vi "turn_back2.vi"(6 "Parâmetros Ini 2":T2={"Gyro Port"=0, "Sensor - Left"=3, "Sensor - Right"=2, "     Color \nSensor Port"=1, "Kp Front"=0.5, "Motor speed"=-15, "Distance to street"=0.0, "Motor speed turns"=16, "Kp Curvas"=0.0} {"Kp Front" format="%.3f"; "Color \nSensor Port" items=["Port 1", "Port 2", "Port 3", "Port 4"]; "Sensor - Right" items=["Port 1", "Port 2", "Port 3", "Port 4"]; "Sensor - Left" items=["Port 1", "Port 2", "Port 3", "Port 4"]; "Gyro Port" items=["Port 1", "Port 2", "Port 3", "Port 4"]}, 8 "NXT/EV3":T1) -> (1 "NXT/EV3 2":T1)   [LabVIEW 2016]
uses:
  <vilib>/NXT/Subs/LVHSConnector.ctl
  <vilib>/NXT/LegoClasses/BrickReference/BrickReference.lvclass
  parametros.ctl
  <vilib>/NXT/Block Support/NXT_InputPort.ctl
  <vilib>/NXT/Block Support/NXT_OutputPort.ctl
  <vilib>/NXT/Dual Mode Library/Sensors/EV3_Gyro_Angle.vi
  <vilib>/NXT/NXTIO Xnodes/NXTIONodeSubVIs/NXTMoveMotors.vi
  <vilib>/NXT/NXTIO Xnodes/NXTIONodeSubVIs/NXTStopMotors.vi
  <vilib>/NXT/NXTIO Xnodes/AddressXNode/NXTIOAddress.xnode
  <vilib>/NXT/NXTIO Xnodes/NXTIOXNode/NXTIO.xnode
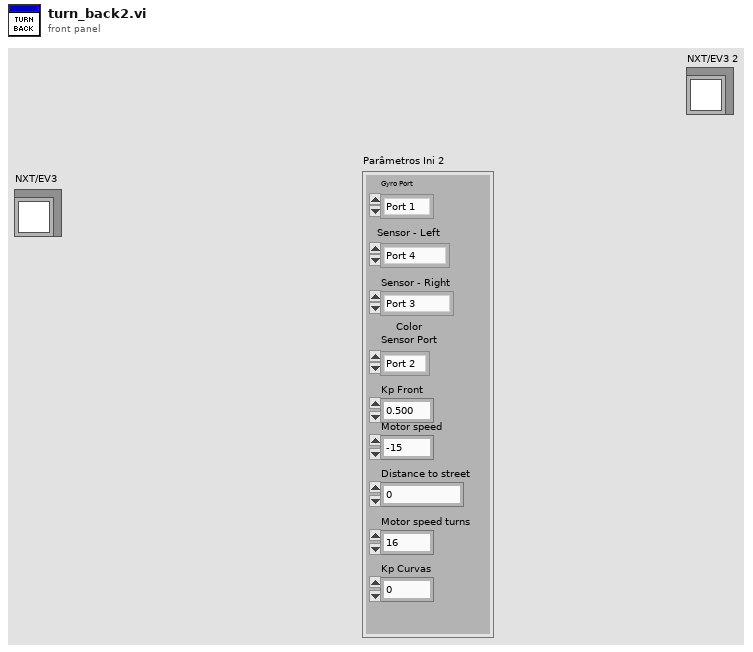
[diagram p1: front panel]
types:
  T1 = typedef "LVHSConnector.ctl" = refnum<class "BrickReference.lvclass">
  T2 = typedef "parametros.ctl" = cluster{"Gyro Port":T3, "Sensor - Left":T3, "Sensor - Right":T3, "     Color \nSensor Port":T3, "Kp Front":dbl, "Motor speed":i32, "Distance to street":dbl, "Motor speed turns":i32, "Kp Curvas":dbl}
  T3 = typedef "NXT_InputPort.ctl" = u32
  T4 = typedef "NXT_OutputPort.ctl" = u8
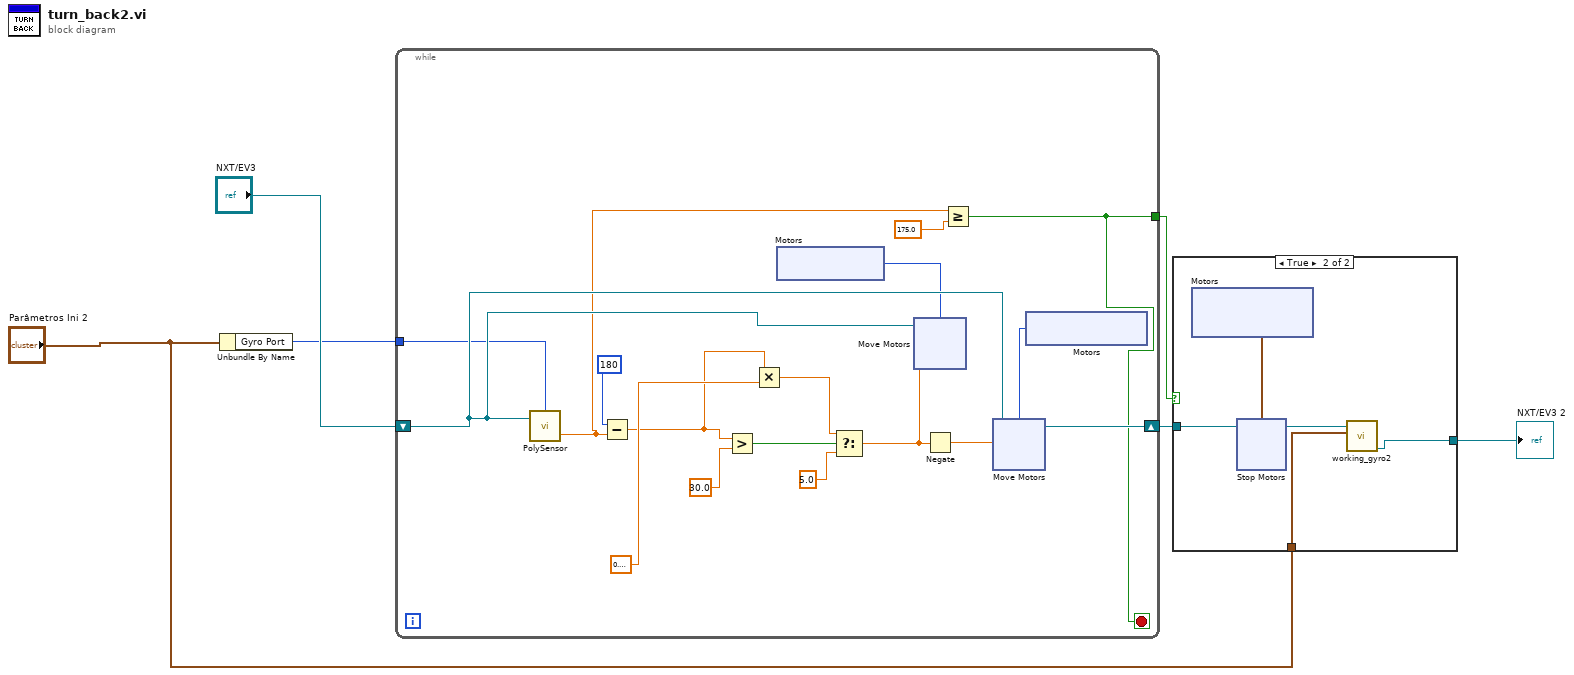
[diagram p0: block diagram]
diagram:
  n1 = Unbundle By Name("Parâmetros Ini 2") -> ("Gyro Port"=w4:T3)
  n2 = while {
    tunnel: w4 -> [w21]
    tunnel: [w7] -> w3
    shift-right: [w23] -> w6
    shift-left: "NXT/EV3" -> [w22]
    stop <- w7 stop-if-true
    n3 = call-poly <vilib>:"PolySensor.vi"("NXT/EV3"=w22, "Port (Port 1)"=w21) -> ("Degrees"=w9:sgl)  [unwired: 1 in, 1 out]
    n4 = Subtract(x=180, y=w9) -> (x-y=w11:sgl)
    n5 = Greater?(x=w11, y=sgl 30.0) -> (0:w16:bool)
    n6 = Multiply(x=w11, y=sgl 0.3) -> (x*y=w10:sgl)
    n7 = xnode "Motors"() -> ("Motor"=w13:T4)
    n8 = Select(t=w10, s=w16, f=sgl 5.0) -> (s? t:f=w14:sgl)
    n9 = xnode "Move Motors"("Power/Speed 1"=w14, "Motors"=w13, "NXT/EV3"=w22) -> ()  [unwired: 1 out]
    n10 = Negate(x=w14) -> (-x=w18:sgl)
    n11 = Greater Or Equal?(x=w9, y=sgl 175.0) -> (x >= y?=w7:bool)
    n12 = xnode "Motors"() -> ("Motor"=w12:T4)
    n13 = xnode "Move Motors"("Power/Speed 1"=w18, "Motors"=w12, "NXT/EV3"=w22) -> ("NXT/EV3"=w23:T1)
  }
  n14 = case shown="True" w3 {
    tunnel: w6 -> [w40 w45]
    tunnel: "Parâmetros Ini 2" -> [_ w42]
    tunnel: [w40 w41] -> w1
    frame False {
    }
    frame True {
      n15 = xnode "Motors"() -> ("Motor"=w44:cluster{"Port":T4, "Port":T4})
      n16 = xnode "Stop Motors"("Motors"=w44, "NXT/EV3"=w45) -> ("NXT/EV3"=w43:T1)
      n17 = call "working_gyro2.vi"("Parâmetros Iniciais"=w42, "NXT/EV3"=w43) -> ("NXT/EV3 2"=w41:T1)  [unwired: 9 in]
    }
  }
  "NXT/EV3 2" <- w1
